vi "Deney-Multi.vi"(1 "f unit":enum16{"mHz", "Hz", "kHz", "MHz", "GHz"}(ring)=enum."kHz", 5 "Frekans":i32(slide)=1 caption="Amplitude(V)" step=1 scale=0.0..100.0, 7 "Amplitude(V)":i32(slide)=20 scale=0.0..20.0, 9 "Teta Aralık":dbl=1.0) -> (6 "Real Matrix":T2)   [LabVIEW 2016]
uses:
  xcontrol/Start Button.xctl
  <vilib>/silver_ctls/ArrayMatrixCluster/Real Matrix NI_Silver.ctl
  <vilib>/Instr/_visa.llb/VISA Configure Serial Port (Instr).vi
  <instrlib>/Tektronix TDS 200 1000 2000 Series/Public/Data/Read (Single Waveform).vi
  <instrlib>/Tektronix TDS 200 1000 2000 Series/Tektronix TDS 200 1000 2000 Series.lvlib
panel:
  in  "Frekans Aralık":dbl=10.0
  in  "Bitir f":dbl=100.0
  in  "Başlat f":dbl=1.0
  in  "polar attributes":T1={"maximum"=0.0, "minimum"=0.0, "clip to min"=FALSE, "log?(F)"=FALSE, "grid color"=6710886, "plot color"=16711680, "fmt and prec"={"format"=enum."Decimal", "precision"=2}, "visible section"=8} {"minimum" format="%0.2f"; "maximum" format="%0.2f"}
  out "XY Graph":cluster{i32[], "Real Matrix":dbl[]}(graph)={[0, 1, 2, 3, 4, 5, 6, 7, 8, 9, 10, 11, 12, 13, 14, 15, 16, 17, 18, 19, 20, 21, 22, 23, 24, 25, 26, 27, 28, 29, 30, 31, 32, 33, 34, 35, 36, 37, 38, 39, 40, 41, 42, 43, 44, 45, 46, 47, 48, 49, 50, 51, 52, 53, 54, 55, 56, 57, 58, 59, 60, 61, 62, 63, 64, 65, 66, 67, 68, 69, 70, 71, 72, 73, 74, 75, 76, 77, 78, 79, 80, 81, 82, 83, 84, 85, 86, 87, 88, 89, 90, 91, 92, 93, 94, 95, 96, 97, 98, 99, 100, 101, 102, 103, 104, 105, 106, 107, 108, 109, 110, 111, 112, 113, 114, 115, 116, 117, 118, 119, 120, 121, 122, 123, 124, 125, 126, 127, 128, 129, 130, 131, 132, 133, 134, 135, 136, 137, 138, 139, 140, 141, 142, 143, 144, 145, 146, 147, 148, 149, 150, 151, 152, 153, 154, 155, 156, 157, 158, 159, 160, 161, 162, 163, 164, 165, 166, 167, 168, 169, 170, 171, 172, 173, 174, 175, 176, 177, 178, 179, 180, 181, 182, 183, 184, 185, 186, 187, 188, 189, 190, 191, 192, 193, 194, 195, 196, 197, 198, 199, 200, 201, 202, 203, 204, 205, 206, 207, 208, 209, 210, 211, 212, 213, 214, 215, 216, 217, 218, 219, 220, 221, 222, 223, 224, 225, 226, 227, 228, 229, 230, 231, 232, 233, 234, 235, 236, 237, 238, 239, 240, 241, 242, 243, 244, 245, 246, 247, 248, 249, 250, 251, 252, 253, 254, 255, 256, 257, 258, 259, 260, 261, 262, 263, 264, 265, 266, 267, 268, 269, 270, 271, 272, 273, 274, 275, 276, 277, 278, 279, 280, 281, 282, 283, 284, 285, 286, 287, 288, 289, 290, 291, 292, 293, 294, 295, 296, 297, 298, 299, 300, 301, 302, 303, 304, 305, 306, 307, 308, 309, 310, 311, 312, 313, 314, 315, 316, 317, 318, 319, 320, 321, 322, 323, 324, 325, 326, 327, 328, 329, 330, 331, 332, 333, 334, 335, 336, 337, 338, 339, 340, 341, 342, 343, 344, 345, 346, 347, 348, 349, 350, 351, 352, 353, 354, 355, 356, 357, 358, 359], "Real Matrix"=[0.9058117558136211, 0.9426152984066833, 0.9381345516903796, 0.9391974627306727, 0.9391310703219856, 0.9371795285402047, 0.9335032861522855, 0.9304365575425565, 0.9307846756772251, 0.9274090074651196, 0.9235150948626124, 0.9242140826074934, 0.9196901138863606, 0.9162864086683812, 0.9082178947467675, 0.911047656143528, 0.9032118635996395, 0.8978063303159379, 0.8981638480310016, 0.8935190056662616, 0.8861748077139071, 0.8790727087161115, 0.8800294659128259, 0.8720891125985217, 0.8644625422369323, 0.8576129138705443, 0.8575497689768316, 0.8492006373529426, 0.8406358566410101, 0.8405837736465182, 0.8295360208046476, 0.8215362176544411, 0.810457002094725, 0.8081045333644754, 0.7996025728061363, 0.7890950917362989, 0.788662671243534, 0.7776275447789194, 0.7628338598899459, 0.7479337302503918, 0.7489913738060436, 0.7376756432212593, 0.7219989520293282, 0.7223134261462048, 0.7072324012621662, 0.6912008463276941, 0.6732526889380832, 0.6766009896723129, 0.6584329003249213, 0.640828263285051, 0.6245417919359195, 0.6240897106479435, 0.6041609011211643, 0.5850747560170694, 0.5854302034525517, 0.5643540408448894, 0.5424407175714369, 0.5211197199562855, 0.520823506111066, 0.49925393550876296, 0.47649404800887574, 0.47676984046292464, 0.4529424819445467, 0.43021720392860224, 0.4057033994638472, 0.4043076023732301, 0.3818221975339064, 0.35882196572843433, 0.35998742750054635, 0.33388740105076603, 0.3101955010153418, 0.28158307426773654, 0.283924711878769, 0.2566059751532502, 0.23072666972132816, 0.20323030396048333, 0.20465075509039415, 0.1787496474585223, 0.1501981876788086, 0.15345247705907455, 0.12390823348638093, 0.09657167696521407, 0.06836353347885694, 0.06818796262630297, 0.047517119999999996, 0.04894263360000001, 0.0495761952, 0.0484448352, 0.05242722239999999, 0.05035508336057849, 0.0517936608, 0.07441450291085813, 0.10335521914256385, 0.10327871972882373, 0.13041941092056566, 0.15343746664359798, 0.18056313263621984, 0.1794974824236721, 0.20480589824118065, 0.2289659589620828, 0.2528429788211244, 0.2532162327692255, 0.2785771988143451, 0.301135924936325, 0.299720714876475, 0.3223535068740002, 0.34642926947189207, 0.3679784716095488, 0.36631775264002353, 0.3865768382651317, 0.40771562130280475, 0.40554379223233794, 0.42765765344157636, 0.449714241256735, 0.4674388201569748, 0.46665591341335716, 0.48434652613515483, 0.5008067182589201, 0.5026310086528976, 0.5194229136664342, 0.5371138847970789, 0.5524425769397725, 0.551189446144586, 0.5669947650405258, 0.5800158625449118, 0.596943626601224, 0.5979843187046553, 0.6101074602942954, 0.6251654629272413, 0.6230539497420688, 0.6382797899476055, 0.6474469771865782, 0.6591861236151793, 0.6592053123982218, 0.6687860898605811, 0.6814931107659646, 0.6802738133146446, 0.6901357209300323, 0.7002262857397644, 0.7091858812125709, 0.7081768315518618, 0.7158400616702599, 0.723418894521829, 0.7233232142780209, 0.7325463657877043, 0.7372526339176628, 0.7467239772498367, 0.7439293349551699, 0.7510823580131556, 0.7590903997025147, 0.762911995586481, 0.7633459168840258, 0.7698328103695048, 0.7740239159752254, 0.7718190936054914, 0.7784472749626611, 0.7823547076778502, 0.7869288938659821, 0.7845130582613086, 0.7900960335158498, 0.7933267053644137, 0.7936813093453882, 0.7974297023687253, 0.8003774211403603, 0.80144197644395, 0.80360925221537, 0.8043902747994175, 0.8071507801137796, 0.8090866959527051, 0.809761908974138, 0.8108437351310606, 0.8134759920656829, 0.8135642438282942, 0.8153790921548144, 0.8169060352514963, 0.8171552373926957, 0.8170990856103086, 0.8180482084001202, 0.818779541859698, 0.8192719870901195, 0.8195692794916573, 0.8208692808390414, 0.8196377370884929, 0.8200311300871435, 0.8178557811682496, 0.8193601218438966, 0.8175522081756196, 0.8157020653551422, 0.8164879851648723, 0.8152192516949711, 0.8157555763632198, 0.813451571283613, 0.8129488292588188, 0.8125686769419559, 0.809979995257749, 0.8079038427813622, 0.8042326756180921, 0.8065390042160322, 0.8022178421495634, 0.7991045362898284, 0.796028226239631, 0.7947027335215948, 0.7909078650369679, 0.7892463778777439, 0.7888984322884679, 0.7829651910745709, 0.7806591612402622, 0.7744988925155162, 0.7743830868933055, 0.7673742919736696, 0.7605272200977838, 0.7620005323851077, 0.7568116520963352, 0.7485024949653487, 0.7413893156779942, 0.7419959407573361, 0.735053115838771, 0.7258826712559172, 0.7269378251820431, 0.7164998155309579, 0.7074935257481089, 0.6969643748908618, 0.6974061863743506, 0.6869336121057522, 0.6753538045317249, 0.663759847172731, 0.6641290187115605, 0.6508366281516016, 0.6395489547186856, 0.6394341995140488, 0.6275679275864259, 0.6113875776803674, 0.5951090755505312, 0.5954548820507707, 0.5817561596605302, 0.5629995284721835, 0.5648743675100829, 0.5471217054358458, 0.5286149198407616, 0.5110932975727674, 0.5139712919287712, 0.4919392302428737, 0.47269112427811594, 0.4728223546414525, 0.45247036154590786, 0.4313034918119647, 0.4097044137847944, 0.4098574639765097, 0.3889339438458797, 0.366528627383536, 0.34398398410739406, 0.3457320418056227, 0.3207748120439545, 0.2974283465600562, 0.2954207700441732, 0.2728904053208129, 0.24607443225106346, 0.21761697466117214, 0.21741474873446093, 0.19189636495478693, 0.16547445219153767, 0.16618673429387815, 0.13763001789480106, 0.10888285696613839, 0.0812515347854542, 0.08210826136881892, 0.052704052474882315, 0.0470193216, 0.0480828, 0.048309072, 0.0484674624, 0.0488973792, 0.0487389888, 0.07600015553653812, 0.10647648760405994, 0.13640418849248315, 0.13541427321257576, 0.1639843034238511, 0.1927985231828867, 0.1942069658256146, 0.22322788658365125, 0.25104188230672964, 0.2827019303201417, 0.28015403831147323, 0.3079384631120034, 0.33502452396405646, 0.3348288159560041, 0.3615430378149064, 0.3886146865777129, 0.41607261406275087, 0.41460586277782246, 0.43826663824208045, 0.464635231973554, 0.46410492027720274, 0.4881777013218986, 0.5118237487411049, 0.5360750135269922, 0.5346191383396572, 0.5595911667593388, 0.5815647527032863, 0.6014625782841935, 0.6017893193733566, 0.6239930948282527, 0.6418047161218764, 0.6441180093207085, 0.6620964441362768, 0.6804056466454744, 0.6978048424738942, 0.6972525134515414, 0.7141405513540375, 0.7322408181197501, 0.7293804734231153, 0.7437998306318019, 0.7603162334042374, 0.7726721834411351, 0.7724648154775859, 0.787831414629664, 0.7995063416513943, 0.7996525383174561, 0.8110511196333454, 0.8230019808730196, 0.8339205040769603, 0.8328947326641223, 0.8430224813206536, 0.8528603279820828, 0.8626337511364468, 0.8641917638682135, 0.8710720213796106, 0.8821396672490401, 0.8801411910015929, 0.885957365145281, 0.8954280649558671, 0.8997592759614638, 0.9011737304354933, 0.9074942304553648, 0.9126045321359431, 0.9152351593392439, 0.9211521812706422, 0.9217013420177107, 0.9274911932816953, 0.9278000486684721, 0.930725645911774, 0.9335617177502908, 0.9398749569851946, 0.9421274284782825, 0.9452089528912292, 0.9483442293885611, 0.9484322568059088, 0.948432423674561, 0.949748985699915, 0.9463165847625051, 0.9524691748406366, 0.9520724698161286, 0.9537459605909023, 0.9527587682519497, 0.9524890810772132, 0.9524191526359799, 0.9519034474029547, 0.9504689502606872, 0.9495797185075024]}
  out "Polar Plot":picture
  out "OSC ERR":bool=TRUE
  out "Out Com":string="x"
  out "İlk Ayar":bool=TRUE
  out "Waveform Data":waveform(dbl)(graph)={"t0"=timestamp(-0.0024999999999999467 s since 1904-01-01), "dt"=2e-06, "Y"=array[2500 elements]}
  in  "Osiloskop Portu":refnum<visa-resource-name>="USB0::0x0699::0x0363::C102985::INSTR"
  in  "Start Button":dbl(xcontrol)
  in  "Reset Dafault":bool
  in  "Teta":u32(slide) scale=0.0..360.0
  in  "Sinyal Jeneratörü Portu":refnum<visa-resource-name>="COM4"
  in  "OUTPUT":bool=TRUE caption="Output"
  in  "cmdOrjin":bool
  in  "cmdStop":bool
  in  "Motor Sürücü Portu":refnum<visa-resource-name>="COM5"
  # "R-O Tarayıcı ile Bilgisayar Kontrollü Halka Anten Radyasyon Paterni Ölçüm Düzeneği Geliştirilmesi"
  # "Teta"
  # "Frekans"
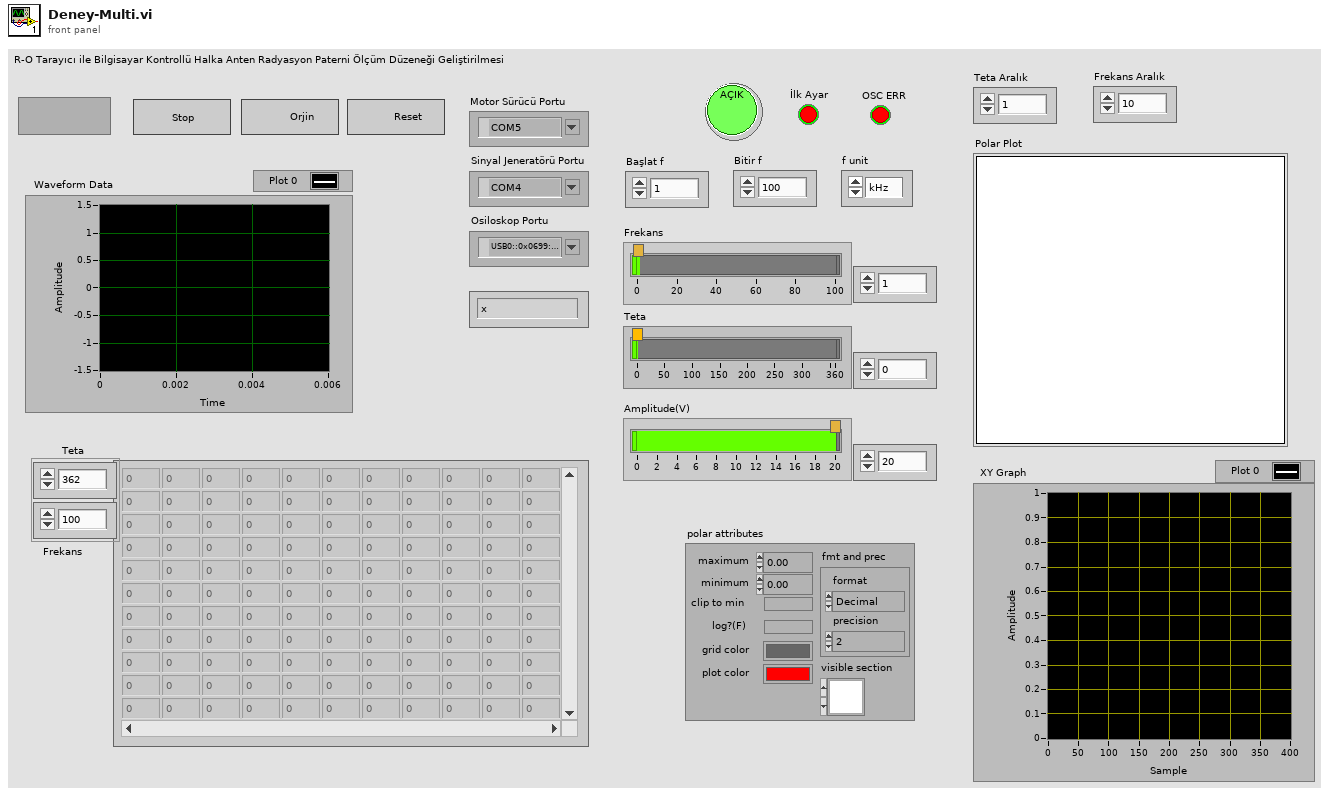
[diagram p1: front panel]
types:
  T1 = cluster{"maximum":dbl, "minimum":dbl, "clip to min":bool, "log?(F)":bool, "grid color":u32, "plot color":u32, "fmt and prec":cluster{"format":enum8{"Decimal", "Scientific", "Engineering", "Binary", "Octal", "Hex"}, "precision":u8}, "visible section":u16}
  T2 = typedef "Real Matrix NI_Silver.ctl" = dbl[][]
  T3 = cluster{"Baud Rate":u32, "Parity":u16, "Stop Bits":u16, "Flow Control":u16}
  T4 = typedef "NI_Matrix.lvlib/RealMatrix.ctl" = dbl[][]
  T5 = typedef "LVBoundsTypeDef.ctl" = cluster{"Width":u32, "Height":u32}
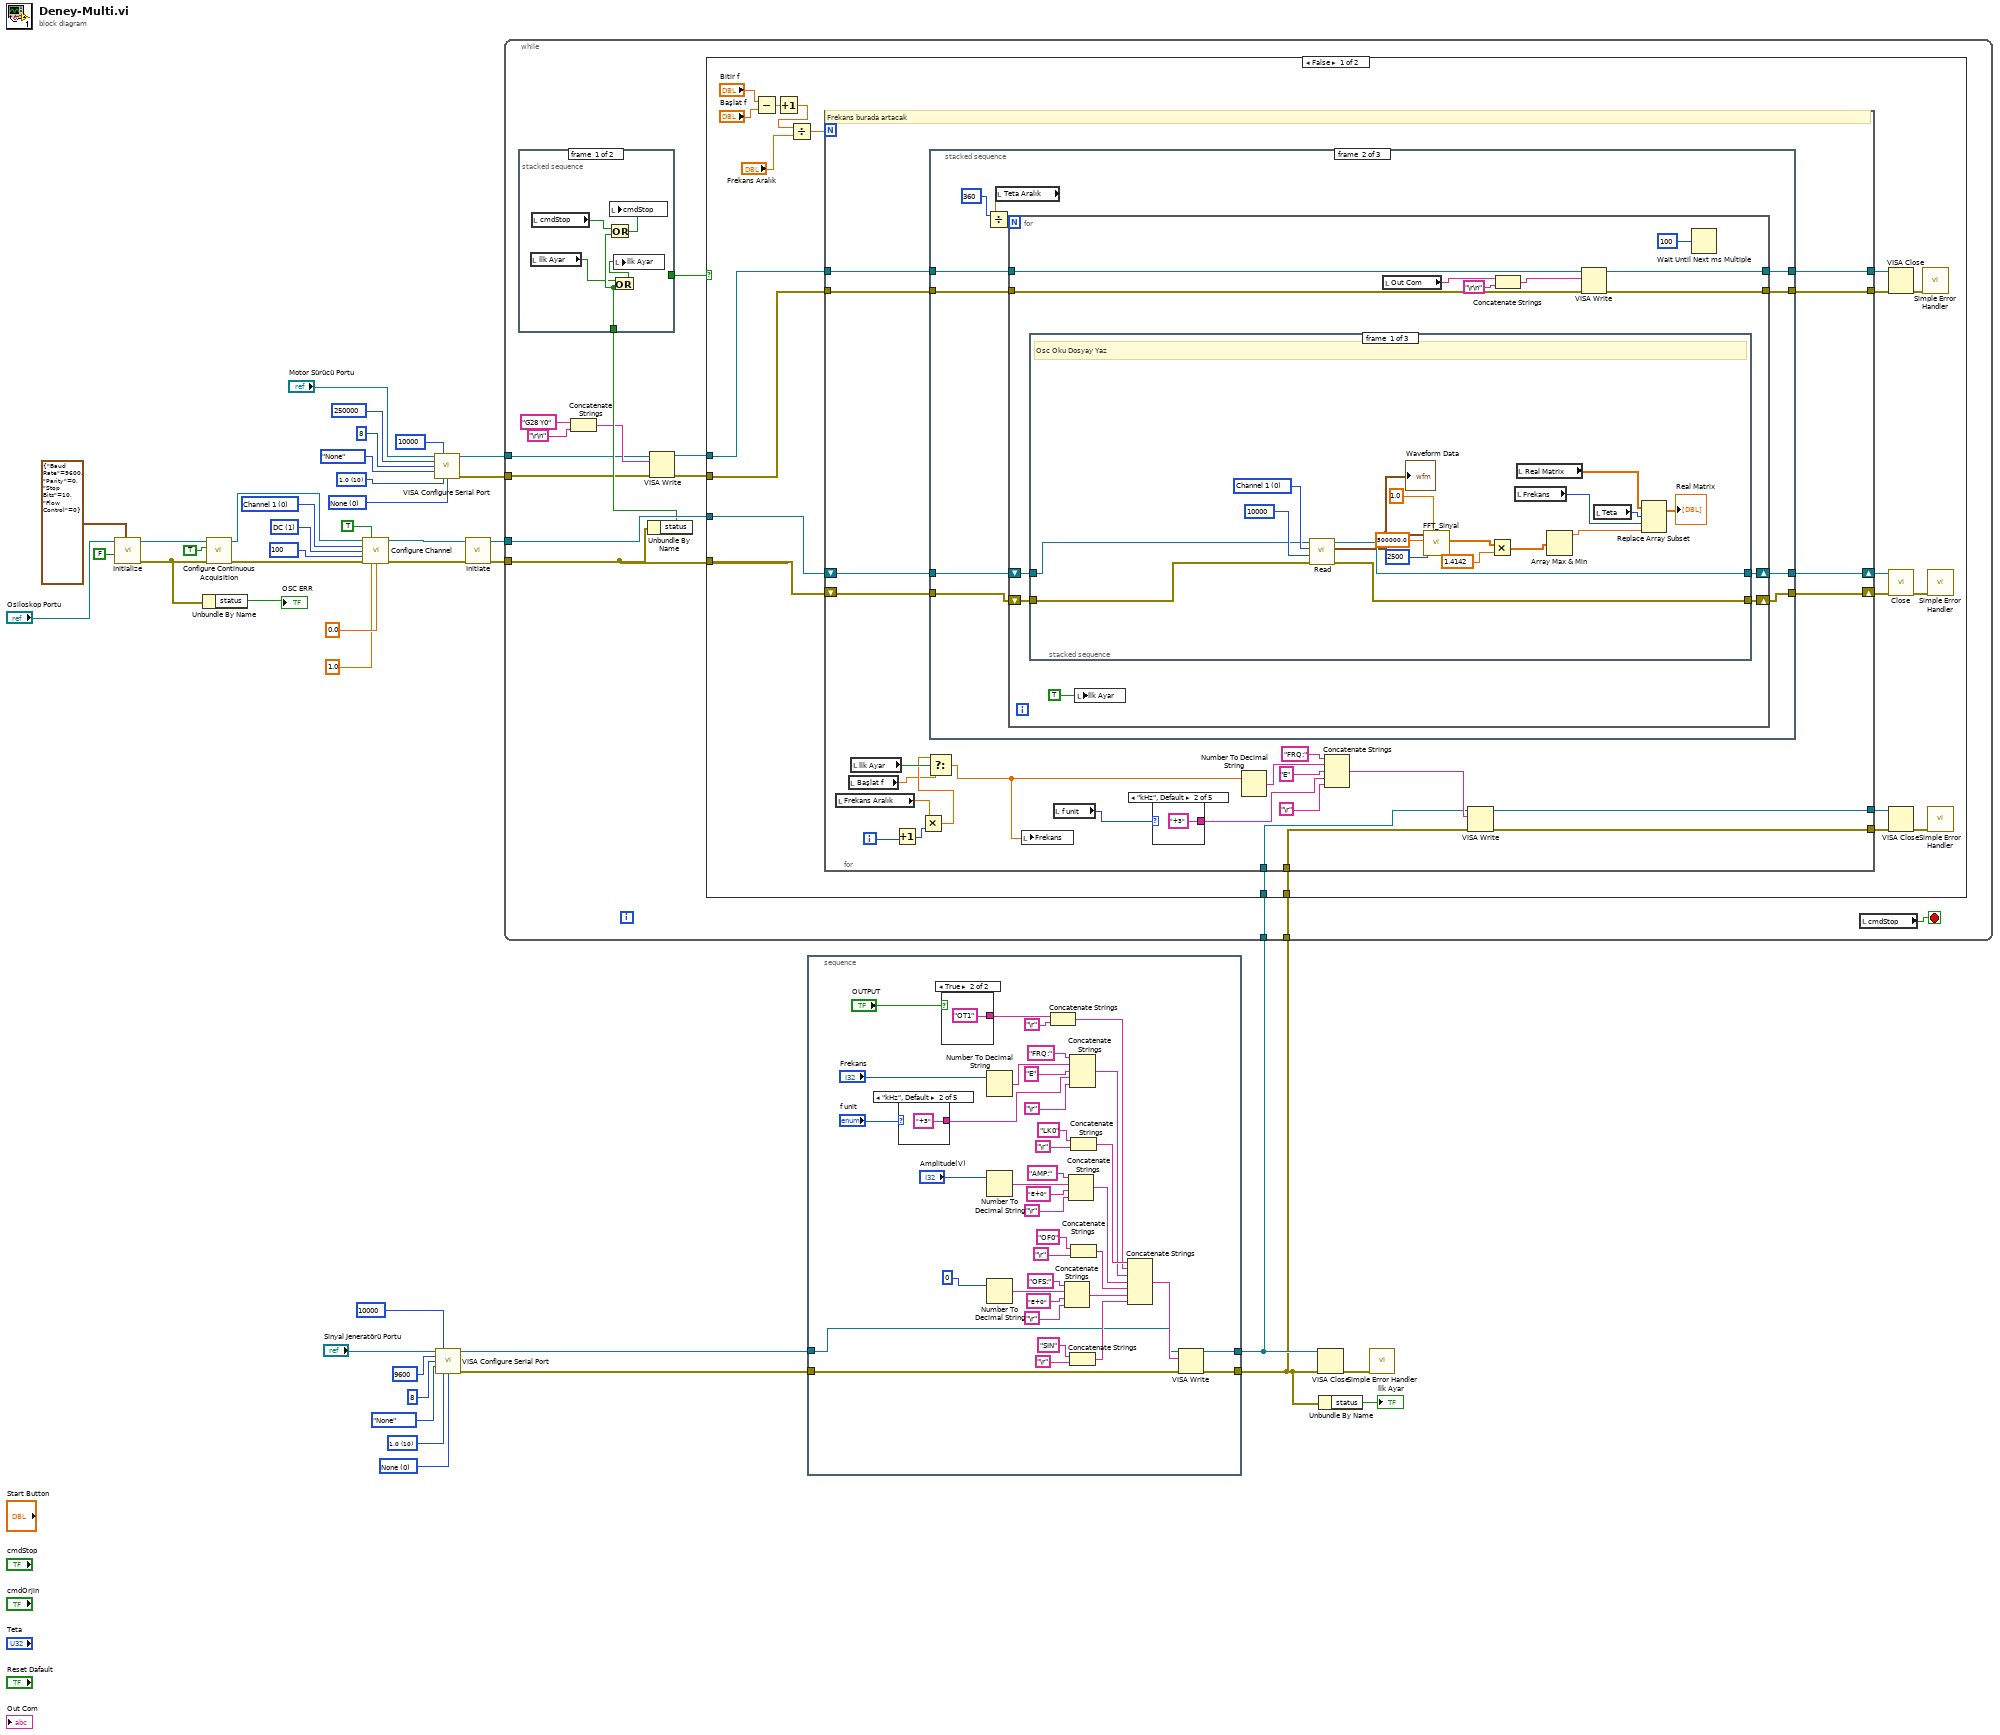
[diagram p0: block diagram]
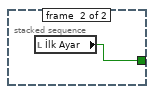
[diagram p2: hidden frame]
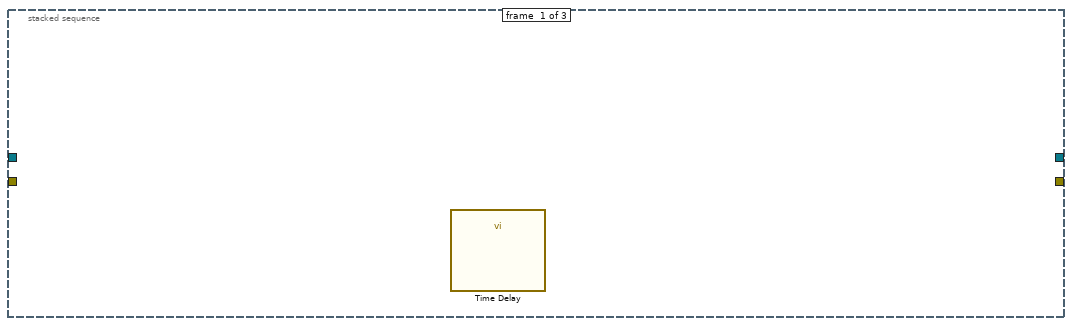
[diagram p3: hidden frame]
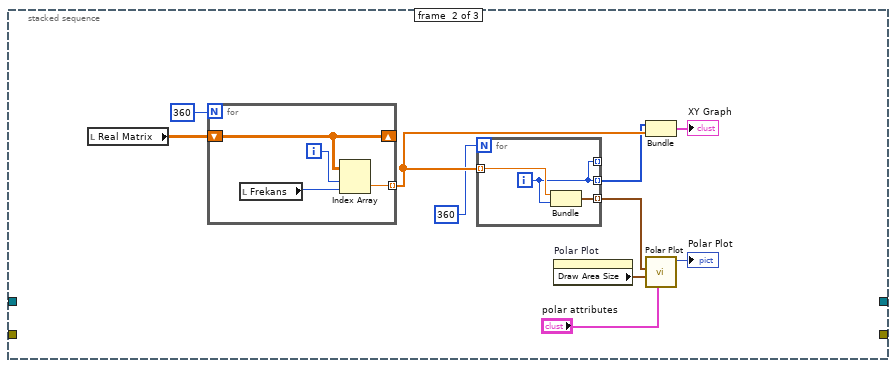
[diagram p4: hidden frame]
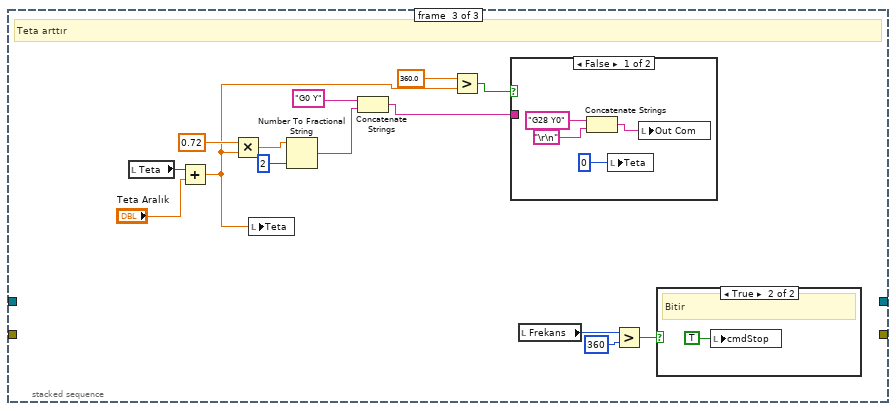
[diagram p5: hidden frame]
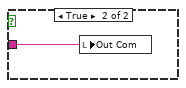
[diagram p6: hidden frame]
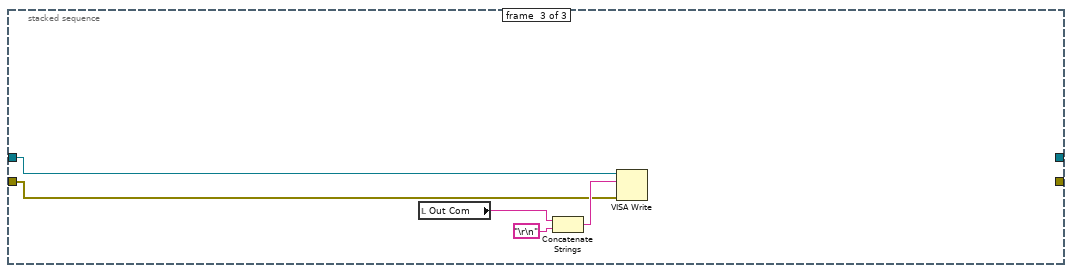
[diagram p8: hidden frame]
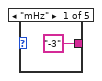
[diagram p9: hidden frame]
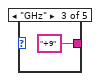
[diagram p10: hidden frame]
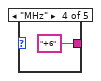
[diagram p11: hidden frame]
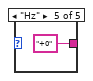
[diagram p12: hidden frame]
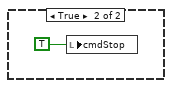
[diagram p13: hidden frame]
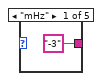
[diagram p14: hidden frame]
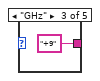
[diagram p15: hidden frame]
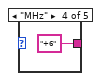
[diagram p16: hidden frame]
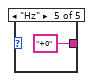
[diagram p17: hidden frame]
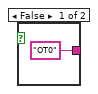
[diagram p18: hidden frame]
diagram:
  w15 = 1 items=["AC", "DC", "Ground"] ("Vertical Coupling (1: DC)")
  w16 = 0 items=["Channel 1", "Channel 2", "Channel 3", "Channel 4", "Math", "Reference A", "Reference B", "Reference C", "Reference D"] ("Channel (0: Channel 1)")
  w18 = 100 items=["1"=1, "10"=10, "20"=20, "50"=50, "100"=100, "500"=500, "1000"=1000] ("Probe Attenuation (10: 10X)")
  w34 = u16 0 items=["None", "XON/XOFF", "RTS/CTS", "XON/XOFF & RTS/CTS", "DTR/DSR", "XON/XOFF & DTR/DSR"] ("flow control (0:none)")
  w33 = u16 10 items=["1.0"=10, "1.5"=15, "2.0"=20] ("stop bits (10: 1 bit)")
  w35 = u16 0 items=["None", "XON/XOFF", "RTS/CTS", "XON/XOFF & RTS/CTS", "DTR/DSR", "XON/XOFF & DTR/DSR"] ("flow control (0:none)")
  w36 = u16 10 items=["1.0"=10, "1.5"=15, "2.0"=20] ("stop bits (10: 1 bit)")
  n1 = call <instrlib>:"Initialize.vi"("Serial Configuration"=T3 {"Baud Rate"=9600, "Parity"=0, "Stop Bits"=10, "Flow Control"=0} ("Osiloskop Config"), "Reset? (T: Yes)"=FALSE, "VISA resource name"="Osiloskop Portu") -> ("error out"=w6:errorcluster, "VISA resource name out"=w7:refnum<visa-resource-name>)  [unwired: 2 in, 5 out]
  n2 = Unbundle By Name(w6) -> ("status"=→"OSC ERR":bool)
  n3 = call <instrlib>:"Configure Continuous Acquisition.vi"("error in (no error)"=w6, "Enable Continuous Acquisition Mode (True)"=TRUE, "VISA resource name"=w7) -> ("error out"=w19:errorcluster, "VISA resource name out"=w22:refnum<visa-resource-name>)  [unwired: 7 out]
  n4 = call <instrlib>:"Configure Channel.vi"("VISA resource name"=w22, "Enable Channel (True)"=TRUE, "Channel (0: Channel 1)"=w16, "Vertical Coupling (1: DC)"=w15, "Probe Attenuation (10: 10X)"=w18, "error in (no error)"=w19, "Vertical Range (10.0 V/div)"=1.0, "Vertical Offset (0.0 divs)"=0.0) -> ("VISA resource name out"=w21:refnum<visa-resource-name>, "error out"=w20:errorcluster)  [unwired: 6 in]
  n5 = call-poly "VISA Configure Serial Port"("VISA resource name"="Motor Sürücü Portu", "timeout (10sec)"=u32 10000, "baud rate (9600)"=u32 250000, "data bits (8)"=u16 8, "parity (0:none)"=enum16{"None", "Odd", "Even", "Mark", "Space"}."None", "stop bits (10: 1 bit)"=w36, "flow control (0:none)"=w35) -> ("VISA resource name out"=w9:refnum<visa-resource-name>, "error out"=w8:errorcluster)  [unwired: 7 in]
  n6 = call-poly "VISA Configure Serial Port"("VISA resource name"="Sinyal Jeneratörü Portu", "timeout (10sec)"=u32 10000, "baud rate (9600)"=u32 9600, "data bits (8)"=u16 8, "parity (0:none)"=enum16{"None", "Odd", "Even", "Mark", "Space"}."None", "stop bits (10: 1 bit)"=w33, "flow control (0:none)"=w34) -> ("VISA resource name out"=w13:refnum<visa-resource-name>, "error out"=w12:errorcluster)  [unwired: 7 in]
  n7 = call <instrlib>:"Initiate.vi"("error in (no error)"=w20, "VISA resource name"=w21) -> ("error out"=w23:errorcluster, "VISA resource name out"=w24:refnum<visa-resource-name>)  [unwired: 8 out]
  n8 = stacked-sequence {
    tunnel: w13 -> [w48]
    tunnel: w12 -> [w47]
    tunnel: [w46] -> w3
    tunnel: [w45] -> w2
    frame #0 {
      n9 = case shown="\"kHz\", Default" "f unit" {
        tunnel: ["-3" "+3" "+9" "+6" "+0"] -> w44
        frame "mHz" {
        }
        frame "kHz", Default {
        }
        frame "GHz" {
        }
        frame "MHz" {
        }
        frame "Hz" {
        }
      }
      n10 = case shown="True" "OUTPUT" {
        tunnel: ["OT0" "OT1"] -> w75
        frame False {
        }
        frame True {
        }
      }
      n11 = Number To Decimal String(number="Frekans") -> (decimal integer string=w70:string)  [unwired: 1 in]
      n12 = Number To Decimal String(number="Amplitude(V)") -> (decimal integer string=w64:string)  [unwired: 1 in]
      n13 = Number To Decimal String(number=0) -> (decimal integer string=w57:string)  [unwired: 1 in]
      n14 = Concatenate Strings(w75, "\r") -> (w72:string)
      n15 = Concatenate Strings("OFS:", w57, "E+0", "\r") -> (w56:string)
      n16 = Concatenate Strings("AMP:", w64, "E+0", "\r") -> (w63:string)
      n17 = Concatenate Strings("FRQ:", w70, "E", w44, "\r") -> (w69:string)
      n18 = Concatenate Strings("SIN", "\r") -> (w55:string)
      n19 = Concatenate Strings("LK0", "\r") -> (w73:string)
      n20 = Concatenate Strings("OF0", "\r") -> (w60:string)
      n21 = Concatenate Strings(w73, w72, w69, w63, w60, w56, w55) -> (w49:string)
      n22 = VISA Write(VISA resource name=w48, write buffer=w49, error in (no error)=w47) -> (VISA resource name out=w46:refnum<visa-resource-name>, error out=w45:errorcluster)  [unwired: 1 out]
    }
  }
  n23 = while {
    tunnel: w24 -> [w100]
    tunnel: w23 -> [w98]
    tunnel: w9 -> [w92]
    tunnel: w8 -> [w89]
    tunnel: w3 -> [w88]
    tunnel: w2 -> [w87]
    stop <- w99 stop-if-true
    n24 = Concatenate Strings("G28 Y0" ("string"), "\r\n") -> (w93:string)
    n25 = Unbundle By Name(w98) -> ("status"=w97:bool)
    n26 = stacked-sequence {
      tunnel: w97 -> [w102 _]
      tunnel: [_ w106] -> w96
      frame #0 {
        n27 = local read "İlk Ayar"() -> (w101:bool)
        n28 = local read "cmdStop"() -> (w104:bool)
        n29 = Or(x=w104, y=w102) -> (x .or. y?=w105:bool)
        n30 = local write "cmdStop"(w105) -> ()
        n31 = Or(x=w101, y=w102) -> (x .or. y?=w103:bool)
        n32 = local write "İlk Ayar"(w103) -> ()
      }
      frame #1 {
        n33 = local read "İlk Ayar"() -> (w106:bool)
      }
    }
    n34 = VISA Write(VISA resource name=w92, write buffer=w93, error in (no error)=w89) -> (VISA resource name out=w91:refnum<visa-resource-name>, error out=w90:errorcluster)  [unwired: 1 out]
    n35 = case shown="False" w96 {
      tunnel: w100 -> [w119 _]
      tunnel: w98 -> [w118 _]
      tunnel: w91 -> [w125 _]
      tunnel: w90 -> [w124 _]
      tunnel: w88 -> [w117 _]
      tunnel: w87 -> [w116 _]
      frame False {
        n36 = Subtract(x="Bitir f", y="Başlat f") -> (x-y=w110:dbl)
        n37 = Increment(x=w110) -> (x+1=w107:dbl)
        n38 = Divide(x=w107, y="Frekans Aralık") -> (x/y=w112:dbl)
        n39 = for {
          N: w112 -> [_]
          shift-right: [w153] -> w127
          shift-left: w119 -> [w147]
          shift-right: [w152] -> w126
          shift-left: w118 -> [w146]
          tunnel: w117 -> [w137]
          tunnel: w116 -> [w138]
          tunnel: [w136] -> w114
          tunnel: [w135] -> w113
          tunnel: w125 -> [w151]
          tunnel: [w149] -> w122
          tunnel: w124 -> [w150]
          tunnel: [w148] -> w121
          i -> [w132]
          # "Frekans burada artacak"
          n40 = local read "Frekans Aralık"() -> (w134:dbl)
          n41 = local read "Başlat f"() -> (w128:dbl)
          n42 = local read "İlk Ayar"() -> (w131:bool)
          n43 = Increment(x=w132) -> (x+1=w133:i32)
          n44 = Multiply(x=w134, y=w133) -> (x*y=w129:dbl)
          n45 = Select(t=w129, s=w131, f=w128) -> (s? t:f=w130:dbl)
          n46 = stacked-sequence {
            tunnel: [_ w164 _] -> w153
            tunnel: [_ w163 _] -> w152
            tunnel: w151 -> [_ w162 w234]
            tunnel: w150 -> [_ w161 w235]
            tunnel: [_ w160 _] -> w149
            tunnel: [_ w159 _] -> w148
            tunnel: w147 -> [_ w158 _]
            tunnel: w146 -> [_ w157 _]
            frame #0 {
              n47 = call "Time Delay"() -> ()  [unwired: 11 in, 1 out]
            }
            frame #1 {
              n48 = local read "Teta Aralık"() -> (w155:dbl)
              n49 = Divide(x=360, y=w155) -> (x/y=w156:dbl)
              n50 = for {
                N: w156 -> [_]
                shift-right: [w175] -> w164
                shift-left: w158 -> [w177]
                shift-right: [w174] -> w163
                shift-left: w157 -> [w176]
                tunnel: w162 -> [w169]
                tunnel: w161 -> [w168]
                tunnel: [w167] -> w160
                tunnel: [w166] -> w159
                n51 = stacked-sequence {
                  tunnel: w177 -> [w187 _ _]
                  tunnel: w176 -> [w186 _ _]
                  tunnel: [w193 _ _] -> w174
                  tunnel: [w192 _ _] -> w175
                  frame #0 {
                    w194 = u16 0 items=["Channel 1", "Channel 2", "Channel 3", "Channel 4", "Math", "Reference A", "Reference B", "Reference C", "Reference D"] ("Channel B (1: Channel 2)")
                    # "Osc Oku Dosyay Yaz"
                    n52 = call-poly <instrlib>:"Read.vi"("error in (no error)"=w186, "Timeout (10000 ms)"=u32 10000 ("Timeout (10000 ms) 2"), "Source (0: Channel 1)"=w194, "VISA resource name"=w187) -> ("error out"=w193:errorcluster, "Waveform Data"=w185:waveform(dbl), "VISA resource name out"=w192:refnum<visa-resource-name>)  [unwired: 5 out]
                    "Waveform Data" <- w185
                    n53 = call "FFT_Sinyal.vi"("Oran"=1.0, "Number of Sample"=2500, "Sampling Frequency"=500000.0, "Sinyal"=w185) -> ("Sinyal Genlik"=w181:dbl[])  [unwired: 2 in, 3 out]
                    n54 = Multiply(x=w181, y=1.4142) -> (x*y=w179:dbl[])
                    n55 = local read "Frekans"() -> (w189:i32)
                    n56 = local read "Real Matrix"() -> (w190:T2)
                    n57 = Array Max & Min(array=w179) -> (max value=w178:dbl)  [unwired: 3 out]
                    n58 = local read "Teta"() -> (w188:u32)
                    n59 = Replace Array Subset ("Set Matrix Elements")(array=w190, new element=w178, index (row)=w188, index (col)=w189) -> (→"Real Matrix":T4)
                  }
                  frame #1 {
                    n60 = local read "Real Matrix"() -> (w205:T2)
                    n61 = for {
                      N: 360 -> [_]
                      shift-right: [w211] -> _
                      shift-left: w205 -> [w211]
                      tunnel: [w212] -> w204 mode=indexing
                      i -> [w210]
                      n62 = local read "Frekans"() -> (w209:i32)
                      n63 = Index Array(array=w211, index (row)=w210, index (col)=w209) -> (element=w212:dbl)
                    }
                    n64 = for {
                      N: 360 -> [_]
                      tunnel: [w207] -> w202 mode=indexing
                      tunnel: [w206] -> _ mode=indexing
                      tunnel: [w206] -> w198 mode=indexing
                      tunnel: w204 -> [w208] mode=indexing
                      i -> [w206]
                      n65 = Bundle("Numeric"=w208, w206) -> (w207:cluster{"Numeric":dbl, i32})  [unwired: 1 in]
                    }
                    n66 = property on="Polar Plot" class="Pict"() -> ("Draw Area Size"=w201:T5)  [unwired: 2 in, 2 out]
                    n67 = Bundle(w198, w204) -> (→"XY Graph":cluster{i32[], dbl[]})  [unwired: 1 in]
                    n68 = call <vilib>:"Polar Plot.vi"("polar attributes"="polar attributes", "dimensions (w,h)"=w201, "data array [mag, phase (deg)]"=w202) -> ("new picture"=→"Polar Plot":picture)  [unwired: 8 in]
                  }
                  frame #2 {
                    # "Teta arttır"
                    n69 = local read "Teta"() -> (w226:u32)
                    n70 = Add(x=w226, y="Teta Aralık") -> (x+y=w216:dbl)
                    n71 = Multiply(x=0.72, y=w216) -> (x*y=w218:dbl)
                    n72 = local write "Teta"(w216) -> ()
                    n73 = Number To Fractional String(number=w218, precision (6)=i16 2) -> (F-format string=w219:string)  [unwired: 2 in]
                    n74 = Concatenate Strings("G0 Y" ("Out Com"), w219) -> (w213:string)
                    n75 = Greater?(x=360.0, y=w216) -> (0:w214:bool)
                    n76 = case shown="False" w214 {
                      tunnel: w213 -> [_ w231]
                      frame False {
                        n77 = Concatenate Strings("G28 Y0" ("string"), "\r\n") -> (w228:string)
                        n78 = local write "Teta"(u32 0 ("Teta")) -> ()
                        n79 = local write "Out Com"(w228) -> ()
                      }
                      frame True {
                        n80 = local write "Out Com"(w231) -> ()
                      }
                    }
                    n81 = local read "Frekans"() -> (w225:i32)
                    n82 = Greater?(x=w225, y=360) -> (0:w223:bool)
                    n83 = case shown="True" w223 {
                      frame False {
                      }
                      frame True {
                        # "Bitir"
                        n84 = local write "cmdStop"(TRUE ("cmdStop")) -> ()
                      }
                    }
                  }
                }
                n85 = local write "İlk Ayar"(TRUE ("İlk Ayar")) -> ()
                n86 = local read "Out Com"() -> (w172:string)
                n87 = Concatenate Strings(w172, "\r\n") -> (w171:string)
                n88 = VISA Write(VISA resource name=w169, write buffer=w171, error in (no error)=w168) -> (VISA resource name out=w167:refnum<visa-resource-name>, error out=w166:errorcluster)  [unwired: 1 out]
                n89 = Wait Until Next ms Multiple(millisecond multiple=u32 100) -> ()  [unwired: 1 out]
              }
            }
            frame #2 {
              n90 = local read "Out Com"() -> (w233:string)
              n91 = Concatenate Strings(w233, "\r\n") -> (w236:string)
              n92 = VISA Write(VISA resource name=w234, write buffer=w236, error in (no error)=w235) -> ()  [unwired: 3 out]
            }
          }
          n93 = local write "Frekans"(w130) -> ()
          n94 = local read "f unit"() -> (w140:enum16{"mHz", "Hz", "kHz", "MHz", "GHz"})
          n95 = case shown="\"kHz\", Default" w140 {
            tunnel: ["-3" "+3" "+9" "+6" "+0"] -> w141
            frame "mHz" {
            }
            frame "kHz", Default {
            }
            frame "GHz" {
            }
            frame "MHz" {
            }
            frame "Hz" {
            }
          }
          n96 = Number To Decimal String(number=w130) -> (decimal integer string=w144:string)  [unwired: 1 in]
          n97 = Concatenate Strings("FRQ:", w144, "E", w141, "\r") -> (w139:string)
          n98 = VISA Write(VISA resource name=w137, write buffer=w139, error in (no error)=w138) -> (VISA resource name out=w135:refnum<visa-resource-name>, error out=w136:errorcluster)  [unwired: 1 out]
        }
        n99 = VISA Close(VISA resource name=w122, error in (no error)=w121) -> (error out=w123:errorcluster)
        n100 = call <instrlib>:"Close.vi"("error in (no error)"=w126, "VISA resource name"=w127) -> ("error out"=w120:errorcluster)  [unwired: 9 in]
        n101 = VISA Close(VISA resource name=w113, error in (no error)=w114) -> (error out=w115:errorcluster)
        n102 = call <vilib>:"Simple Error Handler.vi"("error in (no error)"=w123) -> ()  [unwired: 4 in, 5 out]
        n103 = call <vilib>:"Simple Error Handler.vi"("error in (no error)"=w120) -> ()  [unwired: 4 in, 5 out]
        n104 = call <vilib>:"Simple Error Handler.vi"("error in (no error)"=w115) -> ()  [unwired: 4 in, 5 out]
      }
      frame True {
        n105 = local write "cmdStop"(TRUE ("cmdStop")) -> ()
      }
    }
    n106 = local read "cmdStop"() -> (w99:bool)
  }
  n107 = VISA Close(VISA resource name=w3, error in (no error)=w2) -> (error out=w11:errorcluster)
  n108 = Unbundle By Name(w2) -> ("status"=→"İlk Ayar":bool)
  n109 = call <vilib>:"Simple Error Handler.vi"("error in (no error)"=w11) -> ()  [unwired: 4 in, 5 out]
